vi "fip-trigger_w_cam.vi"() -> ()   [LabVIEW 2022 SP3]
doc: "I. Description:\nThis example demonstrates how to continuously output a waveform using an internal sample clock. The automatic regeneration of data has been disabled, so new data has to be provided throughout the duration of the continuous Analog Output operation. This allows the generation of any arbitrary frequency as this VI computes new data for each iteration of the loop, maintaining phase continuity of the signal.\n\nII. Instructions for Running:\n1. Select the Physical Channel to correspond to where your signal is output on the DAQ device.\n2. Enter the Minimum and Maximum Voltage range.\n3. Specify the desired Sample Clock Rate of the output Waveform. Higher sample clock rates will produce a smoother waveform.\n4. Manually specify the Analog Output buffer size, in number of samples. A larger buffer would help non-regenerative operations avoid errors due to occasional high CPU load. \nNote: \nThe Analog Output buffer has to be at least as big as the amount of data being written to the board per iteration. The recommended buffer size would be at least twice the amount of data being written to the board per iteration.\n5. Enter the Waveform Information. See the documentation of the Basic Function Generator SubVI for information on each parameter.\n\nIII. Block Diagram Steps:\n1. Create an Analog Output Voltage channel.\n2. Configure the task to prohibit the automatic regeneration of data.\n3. Call the DAQmx (Sample Clock) VI to set the sample clock rate. Additionally, set the sample mode to Continuous.\n4. Read the actual sample clock rate (eventually coerced depending on the hardware used). \n5. Compute the desired waveform, using the buffer size and the actual update rate. This VI keeps track of the phase of the waveform to ensure that the generated signal is continuous.\n6. Write the waveform to the output buffer. \n7a. Call the Start VI. This is only needed when the loop is executed for the first time.\n7b. Do nothing.\n8. Loop continuously until user presses the Stop button. Every iteration computes and writes a new waveform to the buffer.\n9. Call the Clear Task VI to clear the Task.\n10. Use the popup dialog box to display an error or warning if any.\n\nIV. I/O Connections Overview:\nMake sure your signal output terminal matches the Physical Channel I/O Control. For further connection information, refer to your hardware reference manual."
uses:
  <vilib>/Utility/error.llb/DialogType.ctl
  <resource>/objmgr/daqmx.rc
  <vilib>/measure/NI_MABase.lvlib
  <vilib>/vision/NI_Vision_Development_Module.lvlib
  <vilib>/DAQmx/configure/timing.llb/DAQmx Timing (Sample Clock).vi
  <vilib>/DAQmx/create/channels.llb/DAQmx Create Channel (AO-Voltage-Basic).vi
  <vilib>/DAQmx/write.llb/DAQmx Write (Analog 1D Wfm NChan NSamp).vi
panel:
  in  "Trigger Mode":u32(ring) items=["Off", "On"]
  out "Iteration #":i32
  out "ROI Overlay":T1(plugin-control)
  in  "Enter File Name":string
  out "Mean":sgl
  in  "Start Recording Data":bool
  in  "Offset 1":dbl=2.5
  in  "Offset 3":dbl=2.5
  in  "Offset 2":dbl=2.5
  in  "Offset 4":dbl=2.5
  in  "Phase 4":dbl=120.0
  in  "Duty Cycle 4":dbl=30.0
  in  "Duty Cycle 3":dbl=30.0
  in  "Duty Cycle 2":dbl=30.0
  in  "Duty Clycle 1":dbl=50.0
  in  "Phase 2":dbl
  in  "Phase 3":dbl=240.0
  in  "Phase 1":dbl=-70.0
  in  "Amplitude 1":dbl=2.5 caption="Amplitude" format="%0.2p"
  in  "Frequency 1":dbl=27.0 caption="Frequency" format="%.2f"
  in  "Waveform Type 1":T2(ring)=enum."Square Wave" caption="Waveform Type"
  in  "CH 1 ON":bool=TRUE
  in  "Amplitude 2":dbl=2.5 caption="Amplitude" format="%0.2p"
  in  "Frequency 2":dbl=9.0 caption="Frequency" format="%.2f"
  in  "Waveform Type 2":T2(ring)=enum."Square Wave" caption="Waveform Type"
  in  "CH 2 ON":bool=TRUE
  in  "CH 4 ON":bool=TRUE
  in  "CH 3 ON":bool=TRUE
  in  "Waveform Type 3":T2(ring)=enum."Square Wave" caption="Waveform Type"
  in  "Frequency 3":dbl=9.0 caption="Frequency" format="%.2f"
  in  "Amplitude 3":dbl=2.5 caption="Amplitude" format="%0.2p"
  in  "Waveform Type 4":T2(ring)=enum."Square Wave" caption="Waveform Type"
  in  "Frequency 4":dbl=9.0 caption="Frequency" format="%.2f"
  in  "Amplitude 4":dbl=2.5 caption="Amplitude" format="%0.2p"
  in  "Size (Samples)":u32=20000
  out "Actual Sample Clock Rate":dbl=20000.0 format="%.2f"
  in  "Sample Clock Rate":dbl=20000.0 format="%0.2f"
  out "Waveform Graph":waveform(dbl)[](graph)=[{"t0"=timestamp(7.25 s since 1904-01-01), "dt"=5e-05, "Y"=array[5000 elements]}, {"t0"=timestamp(7.25 s since 1904-01-01), "dt"=5e-05, "Y"=array[5000 elements]}] caption="Output Waveform"
  in  "Physical Channels":tag="Dev1/ao0:3"
  in  "Minimum Value":dbl=-10.0 format="%0.2f"
  in  "Maximum Value":dbl=10.0 format="%0.2f"
  in  "stop":bool
  # "For instructions, select Help>>Show Context Help"
  # "Channel Parameters"
  # "Timing Parameters"
  # "Waveform Information"
  # "Buffer Parameters"
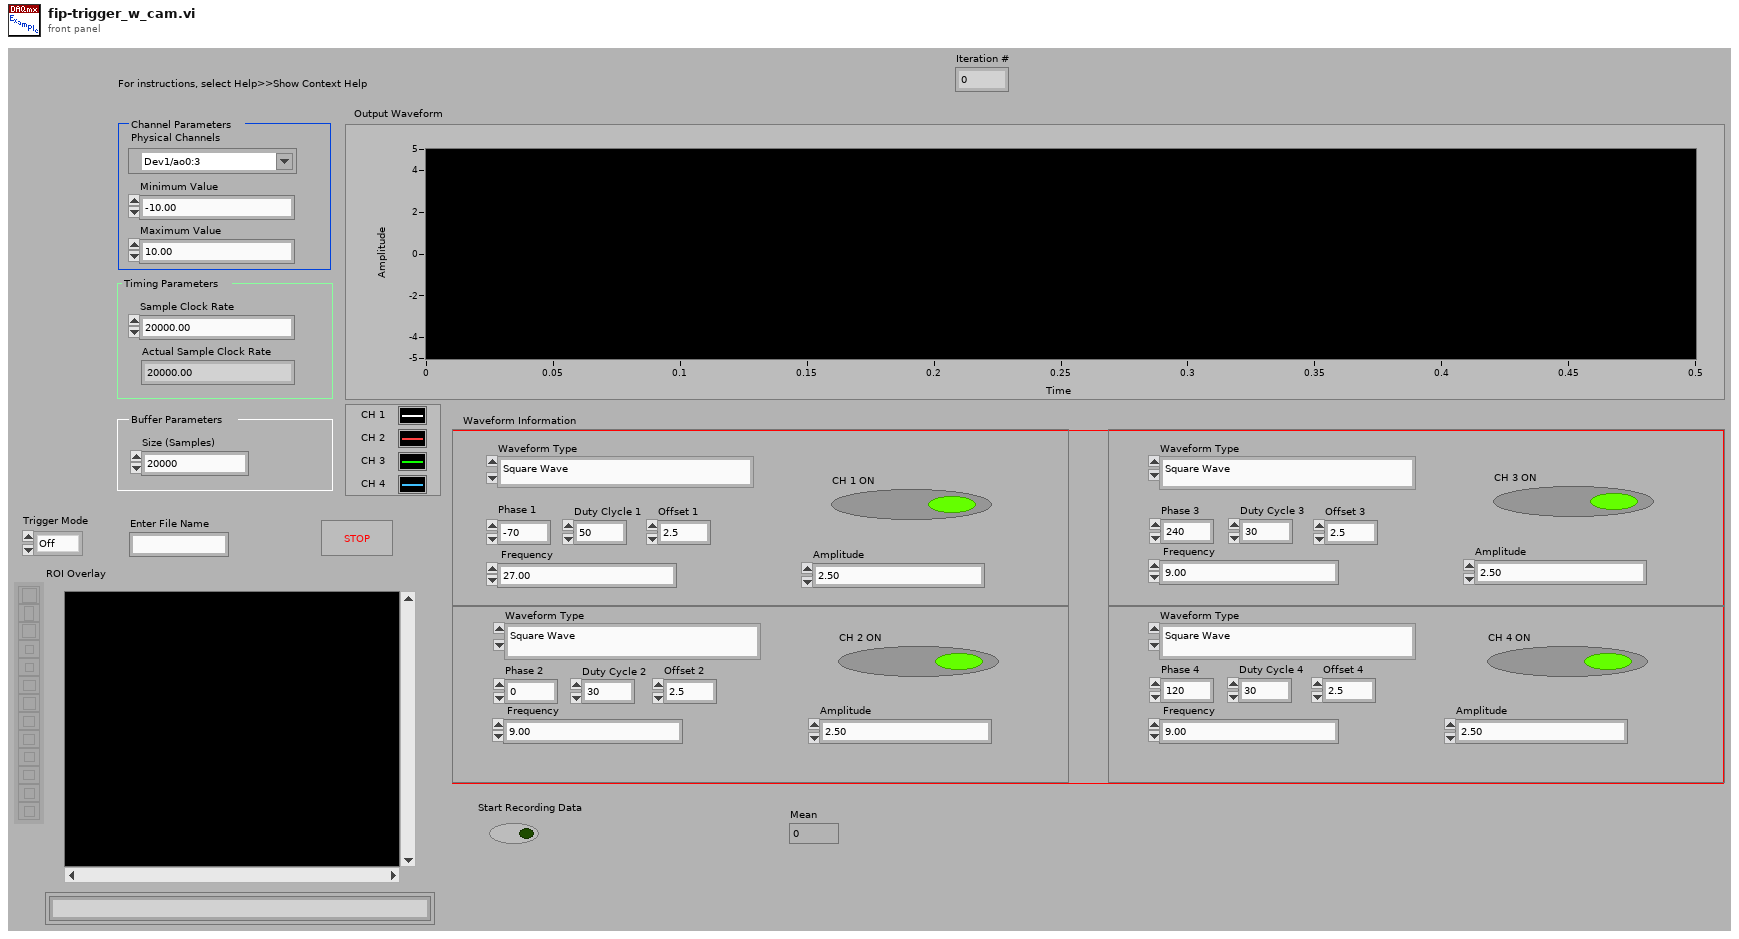
[diagram p1: front panel]
types:
  T1 = typedef "IMAQ Image.ctl" = refnum<image>
  T2 = enum16{"Sine Wave", "Triangle Wave", "Square Wave", "Sawtooth Wave"}
  T3 = typedef "Image Type" = u32
  T4 = typedef "DialogType.ctl" = u16
  T5 = typedef "IMAQ Circle" = cluster{"Center X":i32, "Center Y":i32, "Inner Radius":i32, "Outer Radius":i32, "Start Angle":dbl, "End Angle":dbl}
  T6 = typedef "ROI Descriptor" = cluster{"Global Rectangle":i32[], "Contours":cluster{"ID":enum32{"External", "Internal"}, "Type":u32, "Coordinates":i32[]}[]}
  T7 = cluster{"Min":sgl, "Max":sgl, "Mean":sgl, "Std Dev":sgl, "Count":i32}
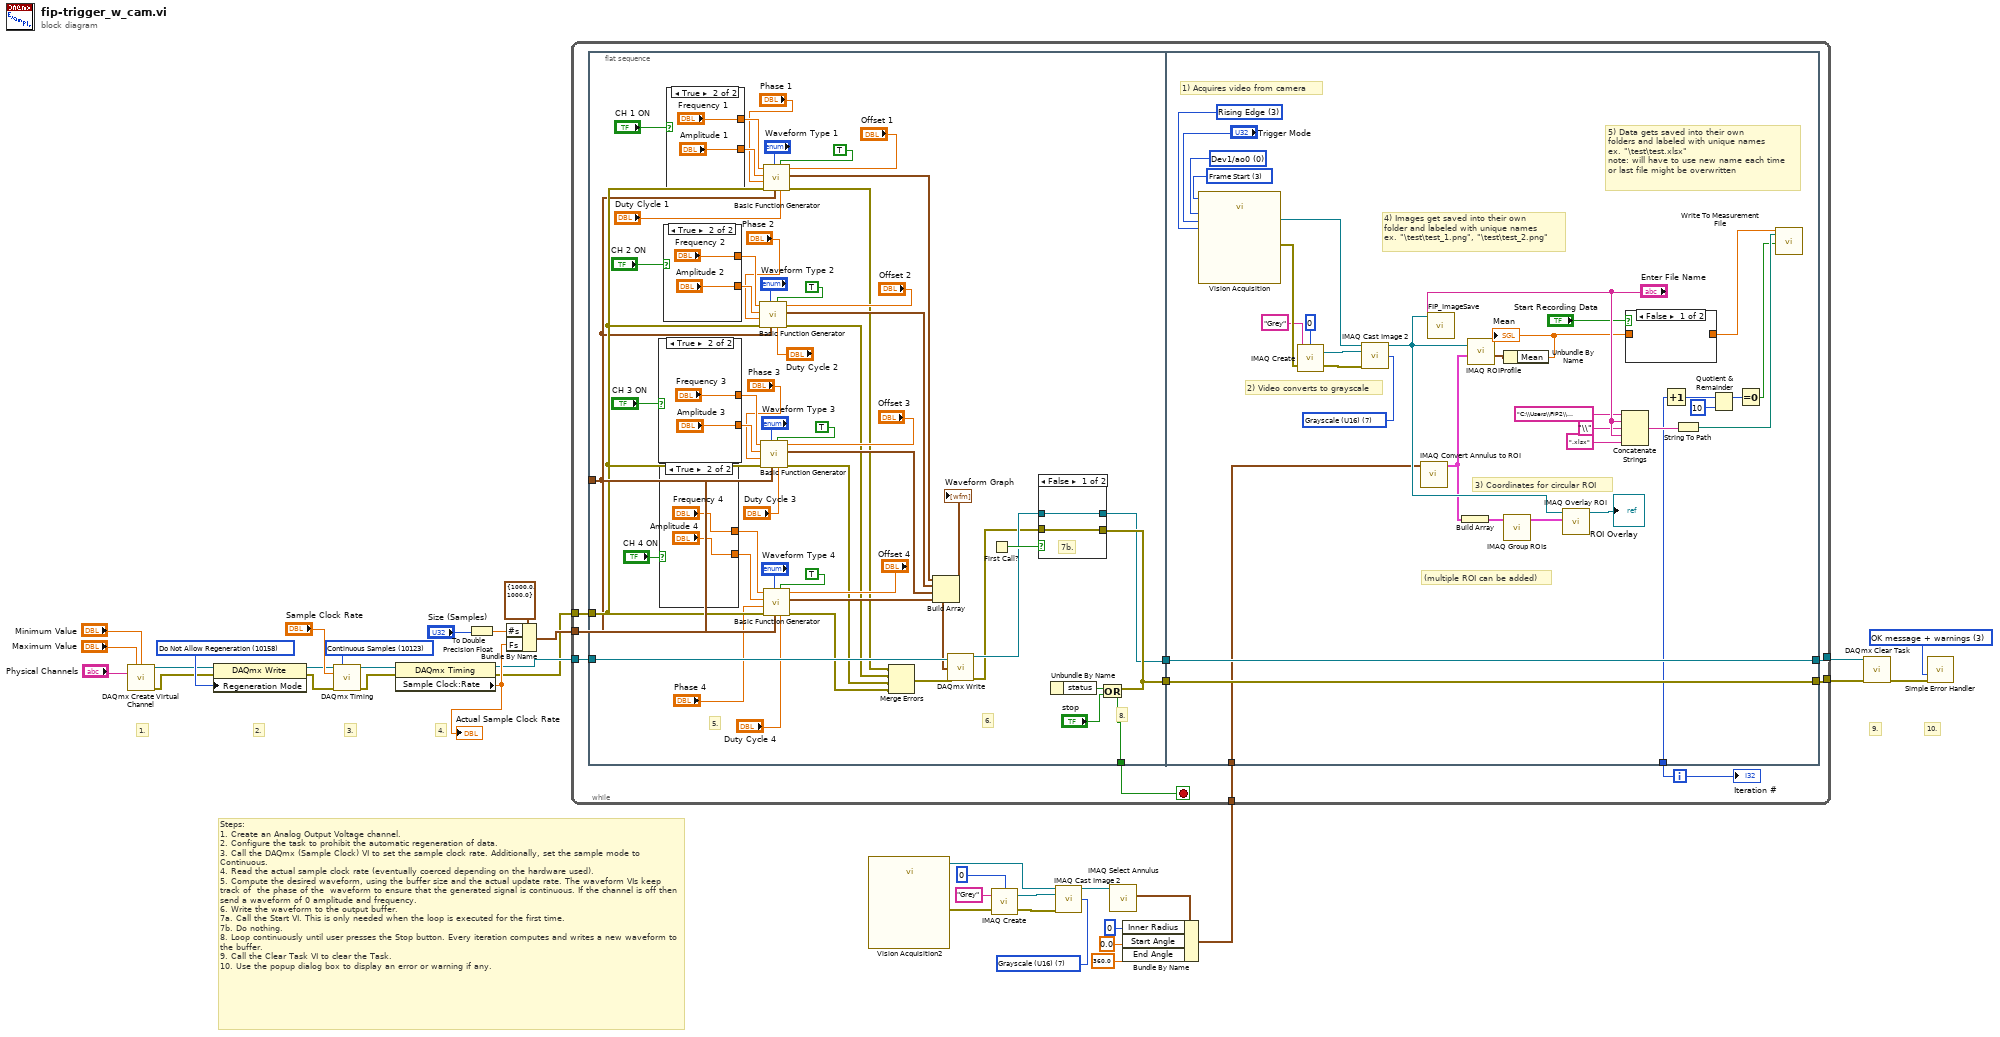
[diagram p0: block diagram]
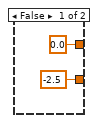
[diagram p2: hidden frame]
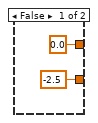
[diagram p3: hidden frame]
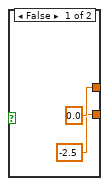
[diagram p4: hidden frame]
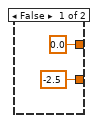
[diagram p5: hidden frame]
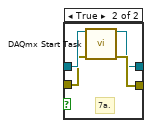
[diagram p6: hidden frame]
diagram:
  w9 = T3 7 items=["Grayscale (U8)", "Grayscale (I16)", "Grayscale (SGL)", "Complex (CSG)", "RGB (U32)", "HSL (U32)", "RGB (U64)", "Grayscale (U16)"] ("Image Type")
  w25 = 10158 items=["Allow Regeneration"=10097, "Do Not Allow Regeneration"=10158] ("RegenMode")
  w34 = T4 3 items=["no dialog", "OK message", "continue or stop message", "OK message + warnings", "continue/stop + warnings"] ("type of dialog (OK msg:1)")
  w35 = 10123 items=["Finite Samples"=10178, "Continuous Samples"=10123] ("sample mode")
  # "4."
  # "3."
  # "Steps:\n1. Create an Analog Output Voltage channel.\n2. Configure the task to prohibit the automatic regeneration of data.\n3. Call the DAQmx (Sample Clock) VI to set the sample clock rate. Additionally, set the sample mode to Continuous.\n4. Read the actual sample clock rate (eventually coerced depending on the hardware used).\n5. Compute the desired waveform, using the buffer size and the actual update rate. The waveform VIs keep track of  the phase of the  waveform to ensure that the generated signal is continuous. If the channel is off then send a waveform of 0 amplitude and frequency.\n6. Write the waveform to the output buffer. \n7a. Call the Start VI. This is only needed when the loop is executed for the first time.\n7b. Do nothing.\n8. Loop continuously until user presses the Stop button. Every iteration computes and writes a new waveform to the buffer.\n9. Call the Clear Task VI to clear the Task.\n10. Use the popup dialog box to display an error or warning if any."
  # "10."
  # "9."
  # "2."
  # "1."
  n1 = call-poly <vilib>:"DAQmx Create Virtual Channel.vi"("maximum value"="Maximum Value", "minimum value"="Minimum Value", "physical channels"="Physical Channels") -> ("task out"=w15:refnum<k21>, "error out"=w14:errorcluster)  [unwired: 6 in, 5 out]
  n2 = property class="DAQmx Write"(reference=w15, error in=w14, "Regeneration Mode"=w25) -> (reference out=w20:refnum<k21>, error out=w19:errorcluster)
  n3 = call-poly <vilib>:"DAQmx Timing.vi"("task/channels in"=w20, "sample mode"=w35, "rate"="Sample Clock Rate", "error in"=w19) -> ("task out"=w30:refnum<k21>, "error out"=w29:errorcluster)  [unwired: 3 in, 7 out]
  n4 = property class="DAQmx Timing"(reference=w30, error in=w29) -> (reference out=w24:refnum<k21>, error out=w23:errorcluster, "Sample Clock:Rate"=w27:dbl)
  "Actual Sample Clock Rate" <- w27
  n5 = To Double Precision Float(number="Size (Samples)") -> (double precision float=w21:dbl)
  n6 = Bundle By Name(cluster=cluster{"Fs":dbl, "#s":dbl} {"Fs"=1000.0, "#s"=1000.0} ("sampling info"), "#s"=w21, "Fs"=w27) -> (w26:cluster{"Fs":dbl, "#s":dbl})
  n7 = call "Vision Acquisition2"() -> ("Image Out"=w7:T1, "error out"=w8:errorcluster)  [unwired: 25 in, 1 out]
  n8 = call "IMAQ Create"("Border Size"=0, "Image Name"="Grey", "error in (no error)"=w8) -> ("New Image"=w13:T1, "error out"=w12:errorcluster)  [unwired: 2 in]
  n9 = call "IMAQ Cast Image 2"("Image Src"=w7, "Image Dst"=w13, "Image Type"=w9, "error in (no error)"=w12) -> ("Image Dst Out"=w6:T1)  [unwired: 10 in, 1 out]
  n10 = call "IMAQ Select Annulus"("Image In"=w6) -> ("Annulus"=w2:T5)  [unwired: 7 in, 3 out]
  n11 = Bundle By Name(cluster=w2, "Inner Radius"=0, "Start Angle"=0.0, "End Angle"=360.0) -> (w1:T5)
  n12 = while {
    tunnel: w24 -> [w45]
    tunnel: [w43] -> w33
    tunnel: w23 -> [w42]
    tunnel: [w44] -> w32
    tunnel: w26 -> [w41]
    tunnel: w1 -> [w37]
    i -> [w38]
    stop <- w46 stop-if-true
    n13 = flat-sequence {
      tunnel: [w99] -> w46
      tunnel: w45 -> [w96]
      tunnel: w42 -> [w76]
      tunnel: w41 -> [w75]
      tunnel: [w95] -> w40
      tunnel: [w94] -> w39
      tunnel: [w154] -> w43
      tunnel: [w155] -> w44
      tunnel: w40 -> [w155]
      tunnel: w39 -> [w154]
      tunnel: w38 -> [w123]
      tunnel: w37 -> [w122]
      frame #0 {
        # "8."
        # "6."
        # "5."
        n14 = case shown="True" "CH 3 ON" {
          tunnel: [-2.5 ("Amplitude 2") "Amplitude 3"] -> w91
          tunnel: [0.0 ("Frequency 2") "Frequency 3"] -> w90
          frame False {
          }
          frame True {
          }
        }
        n15 = case shown="True" "CH 4 ON" {
          tunnel: [-2.5 ("Amplitude") "Amplitude 4"] -> w88
          tunnel: [0.0 ("Frequency") "Frequency 4"] -> w87
          frame False {
          }
          frame True {
          }
        }
        n16 = case shown="True" "CH 2 ON" {
          tunnel: [-2.5 ("Amplitude 2") "Amplitude 2"] -> w83
          tunnel: [0.0 ("Frequency 2") "Frequency 2"] -> w82
          frame False {
          }
          frame True {
          }
        }
        n17 = case shown="True" "CH 1 ON" {
          tunnel: [-2.5 ("Amplitude 2") "Amplitude 1"] -> w79
          tunnel: [0.0 ("Frequency 2") "Frequency 1"] -> w78
          frame False {
          }
          frame True {
          }
        }
        n18 = call <vilib>:"Basic Function Generator.vi"("offset"="Offset 2", "square wave duty cycle (%)"="Duty Cycle 2", "reset signal"=TRUE, "sampling info"=w75, "signal type"="Waveform Type 2", "error in (no error)"=w76, "phase"="Phase 2", "amplitude"=w83, "frequency"=w82) -> ("error out"=w49:errorcluster, "signal out"=w55:waveform(dbl))  [unwired: 1 out]
        n19 = call <vilib>:"Basic Function Generator.vi"("offset"="Offset 3", "square wave duty cycle (%)"="Duty Cycle 3", "reset signal"=TRUE, "sampling info"=w75, "signal type"="Waveform Type 3", "error in (no error)"=w76, "phase"="Phase 3", "amplitude"=w91, "frequency"=w90) -> ("error out"=w48:errorcluster, "signal out"=w54:waveform(dbl))  [unwired: 1 out]
        n20 = call <vilib>:"Basic Function Generator.vi"("offset"="Offset 1", "square wave duty cycle (%)"="Duty Clycle 1", "reset signal"=TRUE, "sampling info"=w75, "signal type"="Waveform Type 1", "error in (no error)"=w76, "phase"="Phase 1", "amplitude"=w79, "frequency"=w78) -> ("error out"=w50:errorcluster, "signal out"=w51:waveform(dbl))  [unwired: 1 out]
        n21 = call <vilib>:"Basic Function Generator.vi"("offset"="Offset 4", "square wave duty cycle (%)"="Duty Cycle 4", "reset signal"=TRUE, "sampling info"=w75, "signal type"="Waveform Type 4", "error in (no error)"=w76, "phase"="Phase 4", "amplitude"=w88, "frequency"=w87) -> ("error out"=w47:errorcluster, "signal out"=w53:waveform(dbl))  [unwired: 1 out]
        n22 = Merge Errors(w50, w49, w48, w47) -> (w56:errorcluster)
        n23 = Build Array(w51, w55, w54, w53) -> (w92:waveform(dbl)[])
        "Waveform Graph" <- w92
        n24 = call-poly <vilib>:"DAQmx Write.vi"("task/channels in"=w96, "data"=w92, "error in"=w56) -> ("task out"=w58:refnum<k21>, "error out"=w57:errorcluster)  [unwired: 1 in, 10 out]
        n25 = First Call?() -> (First Call?: T/F=w93:bool)
        n26 = case shown="False" w93 {
          tunnel: w58 -> [w117 w121]
          tunnel: w57 -> [w116 w120]
          tunnel: [w116 w119] -> w95
          tunnel: [w117 w118] -> w94
          frame False {
            # "7b."
          }
          frame True {
            # "7a."
            n27 = call <vilib>:"DAQmx Start Task.vi"("task/channels in"=w121, "error in"=w120) -> ("task out"=w118:refnum<k21>, "error out"=w119:errorcluster)  [unwired: 12 out]
          }
        }
        n28 = Unbundle By Name(w95) -> ("status"=w98:bool)
        n29 = Or(x=w98, y="stop") -> (x .or. y?=w99:bool)
      }
      frame #1 {
        w125 = u32 0 items=["Dev1/ao0", "Software", "Line 0", "Line 2", "Line 3", "User Output 0", "User Output 1", "User Output 2", "User Output 3", "Counter 0 Start", "Counter 1 Start", "Counter 0 End", "Counter 1 End", "Logic Block 0", "Logic Block 1"] ("Trigger Source")
        w126 = u32 3 items=["Acquisition Start"=2, "Frame Start"=3, "Frame Burst Start"=4] ("Trigger Selector")
        w124 = u32 3 items=["Level Low", "Level High", "Falling Edge", "Rising Edge", "Any Edge"] ("Trigger Activation")
        w127 = T3 7 items=["Grayscale (U8)", "Grayscale (I16)", "Grayscale (SGL)", "Complex (CSG)", "RGB (U32)", "HSL (U32)", "RGB (U64)", "Grayscale (U16)"] ("Image Type")
        # "5) Data gets saved into their own\nfolders and labeled with unique names\nex. \"\\test\\test.xlsx\"\nnote: will have to use new name each time\nor last file might be overwritten"
        # "(multiple ROI can be added)"
        # "4) Images get saved into their own\nfolder and labeled with unique names\nex. \"\\test\\test_1.png\", \"\\test\\test_2.png\""
        # "2) Video converts to grayscale"
        # "3) Coordinates for circular ROI"
        # "1) Acquires video from camera"
        n30 = call "Vision Acquisition"("Trigger Selector"=w126, "Trigger Source"=w125, "Trigger Mode"="Trigger Mode", "Trigger Activation"=w124) -> ("Image Out"=w153:T1, "error out"=w152:errorcluster)  [unwired: 21 in, 1 out]
        n31 = call "IMAQ Create"("Border Size"=0, "Image Name"="Grey", "error in (no error)"=w152) -> ("New Image"=w135:T1, "error out"=w134:errorcluster)  [unwired: 2 in]
        n32 = call "IMAQ Cast Image 2"("Image Src"=w153, "Image Dst"=w135, "Image Type"=w127, "error in (no error)"=w134) -> ("Image Dst Out"=w150:T1)  [unwired: 10 in, 1 out]
        n33 = call "IMAQ Convert Annulus to ROI"("Annulus"=w122) -> ("ROI Descriptor"=w137:T6)  [unwired: 8 in, 1 out]
        n34 = call "FIP_ImageSave.vi"("File Name"="Enter File Name", "Image"=w150) -> ()  [unwired: 10 in]
        n35 = Build Array(w137) -> (w138:T6[])
        n36 = call "IMAQ ROIProfile"("ROI Descriptor"=w137, "Image"=w150) -> ("ROI Pixel Statistics"=w136:T7)  [unwired: 2 in, 4 out]
        n37 = Unbundle By Name(w136) -> ("Mean"=w144:sgl)
        "Mean" <- w144
        n38 = call "IMAQ Group ROIs"("ROI Descriptors"=w138) -> ("ROI Descriptor out"=w139:T6)  [unwired: 3 in, 1 out]
        n39 = call "IMAQ Overlay ROI"("ROI Descriptor"=w139, "Image"=w150) -> ("Image Out"=→"ROI Overlay":T1)  [unwired: 8 in, 1 out]
        n40 = Concatenate Strings("C:\\Users\\FIP2\\Documents\\Labview Photos\\" ("string"), "Enter File Name", "\\" ("string"), "Enter File Name", ".xlsx" ("string")) -> (w140:string)
        n41 = case shown="False" "Start Recording Data" {
          tunnel: w144 -> [_ w156]
          tunnel: [_ w156] -> w146
          frame False {
          }
          frame True {
          }
        }
        n42 = Increment(x=w123) -> (x+1=w142:i32)
        n43 = String To Path(string=w140) -> (path=w148:path)
        n44 = Quotient & Remainder(x=w142, y=10) -> (x-y*floor(x/y)=w141:i32)  [unwired: 1 out]
        n45 = Equal To 0?(x=w141) -> (x = 0?=w147:bool)
        n46 = call "Write To Measurement File"("Signals"=w146, "Flush? (T)"=w147, "Filename"=w148) -> ()  [unwired: 14 in, 3 out]
      }
    }
    "Iteration #" <- w38
  }
  n47 = call <vilib>:"DAQmx Clear Task.vi"("task in"=w33, "error in"=w32) -> ("error out"=w36:errorcluster)  [unwired: 13 out]
  n48 = call <vilib>:"Simple Error Handler.vi"("type of dialog (OK msg:1)"=w34, "error in (no error)"=w36) -> ()  [unwired: 8 out]
